vi "2810A Parse Scan List.vi"(11 "Matrix Input String":string="[c2->card1r2->c26], [c3->card1r3->c27]; [c6->card1r2->c26], [c7->card1r3->c27]; [c10->card1r2->c26], [c11->card1r3->c27]; [c14->card1r2->c26], [c15->card1r3->c27]; [c18->card1r2->c26], [c19->card1r3->c27]; [c22->card1r2->c26], [c23->card1r3->c27];") -> (3 "Channel Array":string[](array[string]))   [LabVIEW 2019, in "SupportVIs.lvlib"]
uses:
  SupportVIs.lvlib
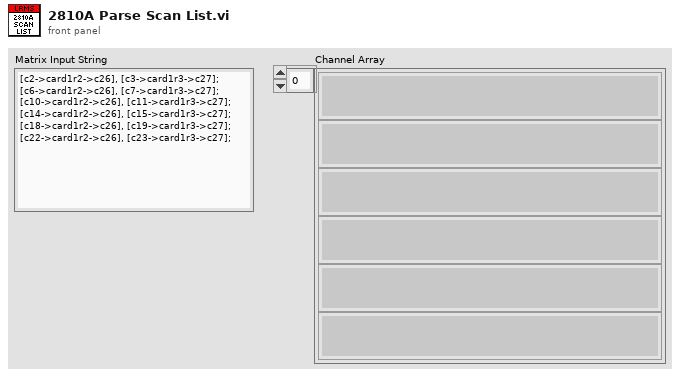
[diagram p1: front panel]
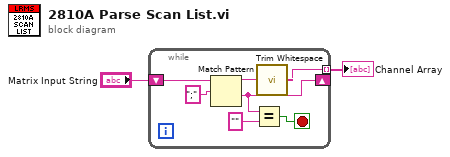
[diagram p0: block diagram]
diagram:
  n1 = while {
    tunnel: [w3] -> w1 mode=indexing
    shift-right: [w5] -> _
    shift-left: "Matrix Input String" -> [w8]
    stop <- w7 stop-if-true
    n2 = Match Pattern(string=w8, regular expression=";" ("search string")) -> (before substring=w4:string, after substring=w5:string)  [unwired: 1 in, 2 out]
    n3 = Equal?(x=w5, y="") -> (x = y?=w7:bool)
    n4 = call <vilib>:"Trim Whitespace.vi"("string"=w4) -> ("trimmed string"=w3:string)  [unwired: 1 in]
  }
  "Channel Array" <- w1
